vi "Main.vi"(8 "error in (no error)":errorcluster) -> ()   [LabVIEW 2017, in "EventModule.lvlib"]
uses:
  EventModule.lvlib
  <userlib>/NIST/ModuleAdminLib/ModuleAdmin/ModuleAdmin.lvclass
  C:/Program Files (x86)/National Instruments/LabVIEW 2017/user.lib/NIST/ModuleAdminLib/ModuleAdminBase/ModuleAdminBase.lvclass
  PublicAPI/Arguments/Requests/clStopArgument.ctl
  EventPlugins/EventPluginBaseClass/EventPluginBaseClass.lvclass
  C:/Program Files (x86)/National Instruments/LabVIEW 2017/user.lib/NIST/BaseClasses/BasePlugin_class/BasePlugin.lvclass
  <userlib>/NIST/ModuleAdminLib/ModuleAdmin/ModuleAdmin.lvclass/ModuleAdmin.ctl
  <userlib>/NIST/BaseClasses/BasePlugin_class/BasePlugin.lvclass/BasePlugin.ctl
  EventPlugins/EventPluginBaseClass/TypeDefs/clEvtConfig.ctl
  PublicAPI/Arguments/Requests/dblTimeArray.ctl
  PublicAPI/Arguments/Requests/dblEvtParams.ctl
  EventPlugins/EventPluginBaseClass/EventPluginBaseClass.lvclass/EventPluginBaseClass.ctl
  <vilib>/Utility/error.llb/DialogType.ctl
  <userlib>/NIST/ModuleAdminLib/ModuleAdmin/Accessors/Read ShowPanel_.vi
  <userlib>/NIST/ModuleAdminLib/ModuleAdmin/Accessors/Write ShowPanel_.vi
  <userlib>/NIST/BaseClasses/BasePlugin_class/Accessors/Write PluginIniFilePath.vi
  <userlib>/NIST/BaseClasses/BasePlugin_class/Accessors/Read PluginIniFilePath.vi
  EventPlugins/EventPluginBaseClass/Accessors/Write BusNumber.vi
  EventPlugins/EventPluginBaseClass/Accessors/Read BusNumber.vi
  <userlib>/NIST/ModuleAdminLib/ModuleAdmin/Accessors/Read CloneRegRef.vi
  <vilib>/Utility/error.llb/Error Cluster From Error Code.vi
  EventPlugins/EventPluginBaseClass/Accessors/Write EvtConfig.vi
  EventPlugins/EventPluginBaseClass/Accessors/Read EvtConfig.vi
  <vilib>/Analysis/1siggen.llb/Ramp Pattern by Delta.vi
  EventPlugins/EventPluginBaseClass/Accessors/Read TimeArray.vi
  EventPlugins/EventPluginBaseClass/Accessors/Read EvtParams.vi
  <vilib>/ErrorRing/Error Ring.xnode
  <userlib>/NIST/ModuleAdminLib/CloneRegistration/CloneRegistration.lvclass
  <userlib>/NIST/ModuleAdminLib/ModuleAdmin.lvlib
  <userlib>/NIST/BaseClasses/Object_class/BaseObject.lvclass
  <vilib>/Analysis/NI_AALBase.lvlib
panel:
  out "error out":errorcluster
  in  "ModuleAdmin":refnum<class "ModuleAdmin.lvclass">
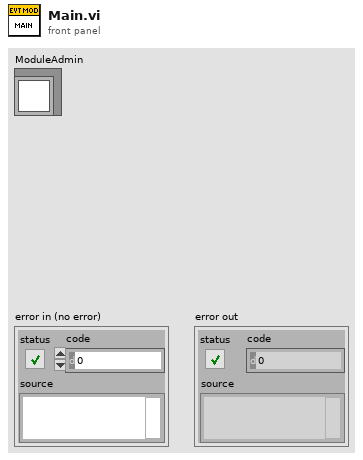
[diagram p1: front panel]
types:
  T1 = typedef "EventModule.lvlib/clRequestEvents.ctl" = cluster{"StopRequest":refnum<user-event>, "LoadPluginRequest":refnum<user-event>, "WriteEvtConfig":refnum<user-event>, "ReadEvtConfig":refnum<user-event>, "WriteTimeArray":refnum<user-event>, "ReadTimeArray":refnum<user-event>, "WriteEvtParams":refnum<user-event>, "ReadEvtParams":refnum<user-event>, "GetEvtReportArray":refnum<user-event>, "ReadPathToPlugin":refnum<user-event>, "GetEvtSignal":refnum<user-event>, "WriteBusNumber":refnum<user-event>, "ReadBusNumber":refnum<user-event>, "ShowPanel":refnum<user-event>}
  T2 = typedef "EventModule.lvlib/clBroadcastEvents.ctl" = cluster{"DidInit":refnum<user-event>, "StatusUpdate":refnum<user-event>, "ErrorReport":refnum<user-event>, "DidStop":refnum<user-event>, "ReadEvtConfig":refnum<user-event>, "ReadTimeArray":refnum<user-event>, "ReadEvtParams":refnum<user-event>, "GetEvtReportArray":refnum<user-event>, "ReadPathToPlugin":refnum<user-event>, "GetEvtSignal":refnum<user-event>, "ReadBusNumber":refnum<user-event>}
  T3 = typedef "EventModule.lvlib/clStopArgument.ctl" = cluster{"Exit via Stop Module Req?":bool, "Wait for Module to stop?":bool, "ModuleAdmin":refnum<class "ModuleAdmin.lvclass">}
  T4 = enum32{"Invalid", "Standard", "Closed", "Hidden", "Minimized", "Maximized"}
  T5 = typedef "EventPlugins.lvlib/EventPluginBaseClass.lvclass/clEvtConfig.ctl" = cluster{"T0(UTC)":dbl, "F0":dbl, "Fs":i32, "FSamp":u32, "bPosSeq":bool}
  T6 = typedef "EventModule.lvlib/dblTimeArray.ctl" = dbl[]
  T7 = typedef "EventModule.lvlib/dblEvtParams.ctl" = dbl[][]
  T8 = typedef "EventPlugins.lvlib/EventPluginBaseClass.lvclass/clEvtReportArray.ctl" = T9[]
  T9 = typedef "EventPlugins.lvlib/EventPluginBaseClass.lvclass/clEvtReport.ctl" = cluster{"Timestamp":dbl, "Synx":cdb[], "Freq":dbl, "ROCOF":dbl, "ID":i16}
  T10 = typedef "EventPlugins.lvlib/EventPluginBaseClass.lvclass/dblEvtSignalArray.ctl" = dbl[][]
  T11 = typedef "DialogType.ctl" = u16
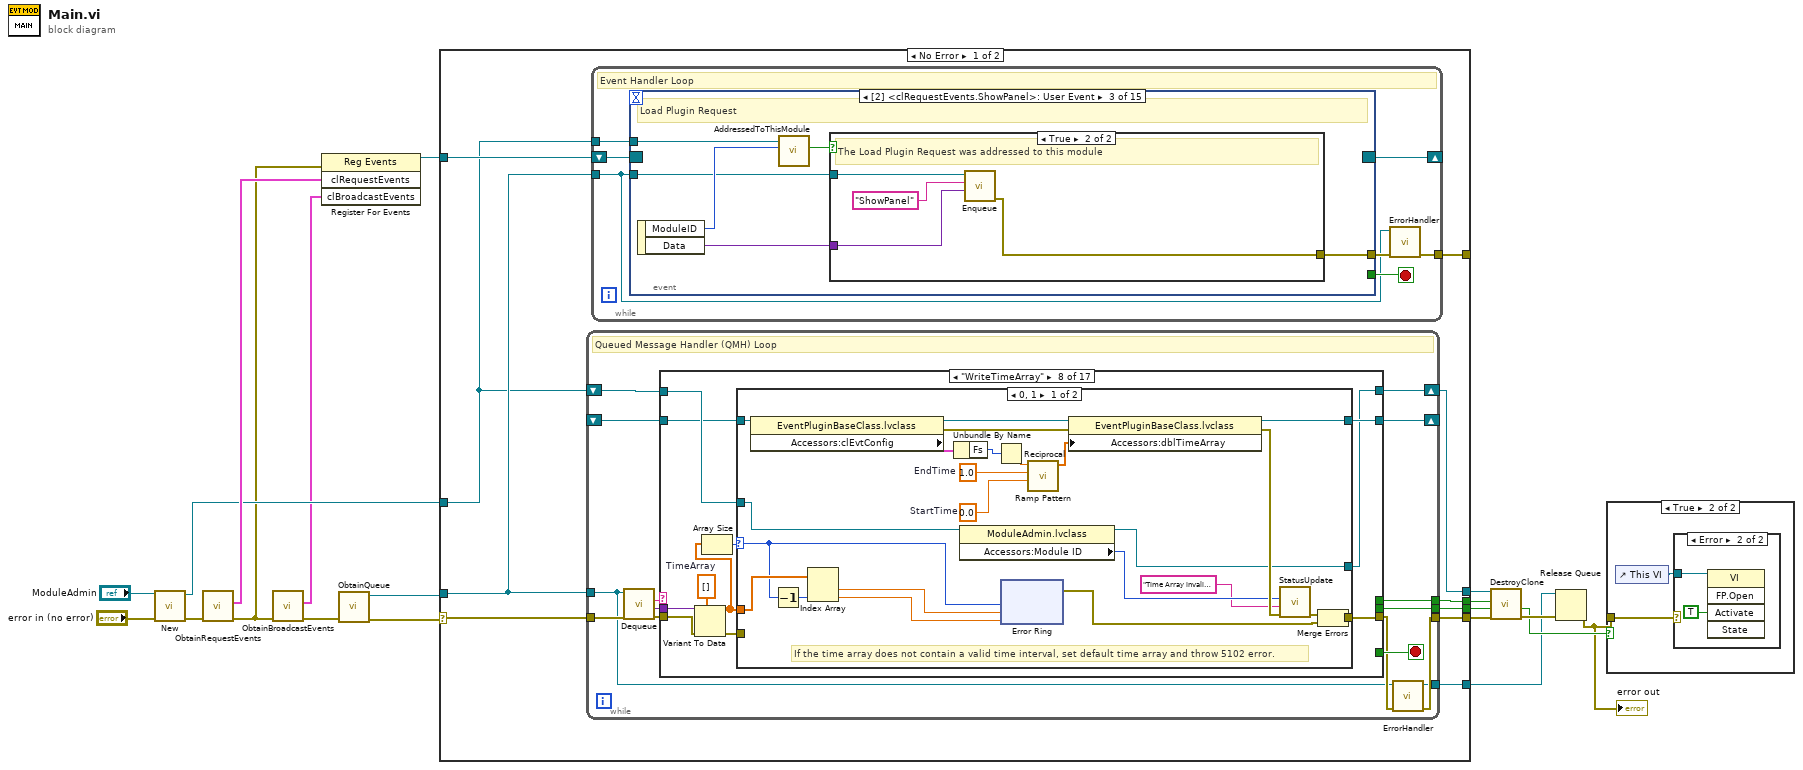
[diagram p0: block diagram]
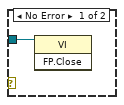
[diagram p3: hidden frame]
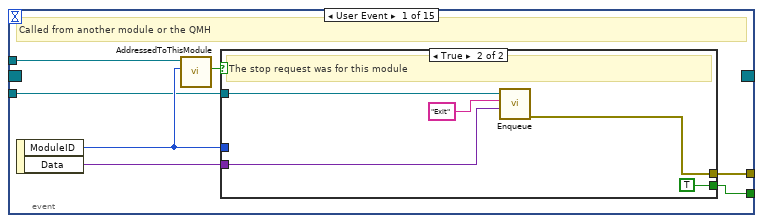
[diagram p4: hidden frame]
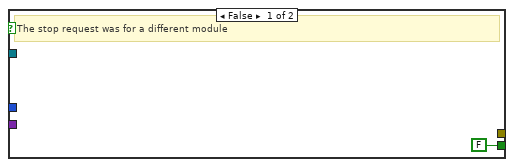
[diagram p5: hidden frame]
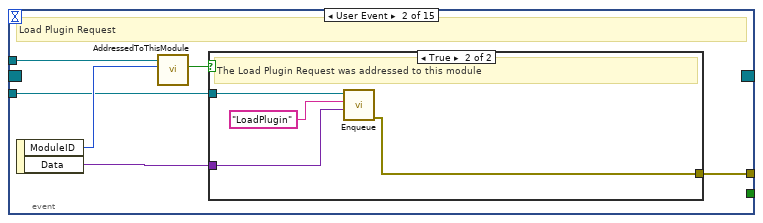
[diagram p6: hidden frame]
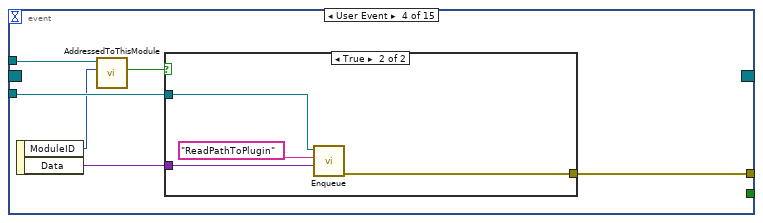
[diagram p9: hidden frame]
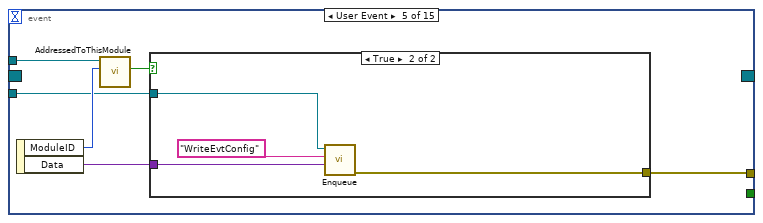
[diagram p11: hidden frame]
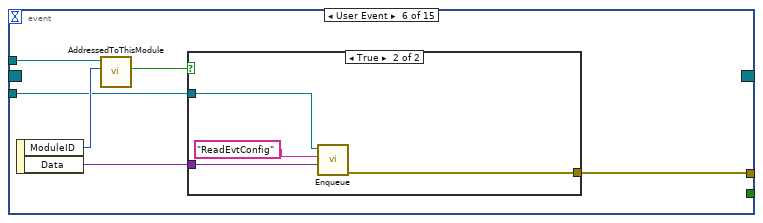
[diagram p13: hidden frame]
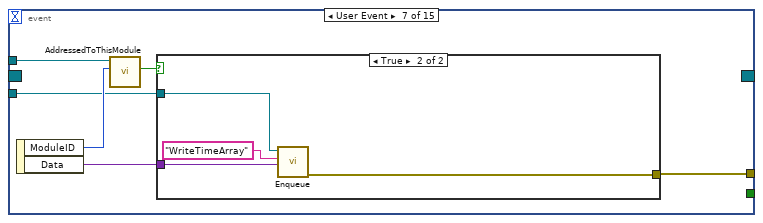
[diagram p15: hidden frame]
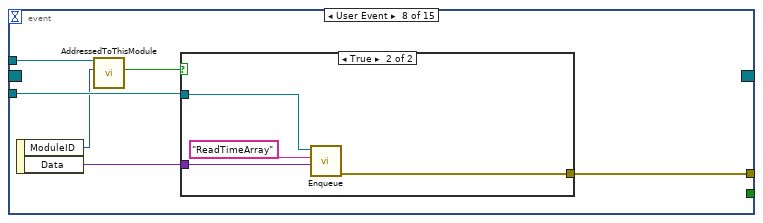
[diagram p17: hidden frame]
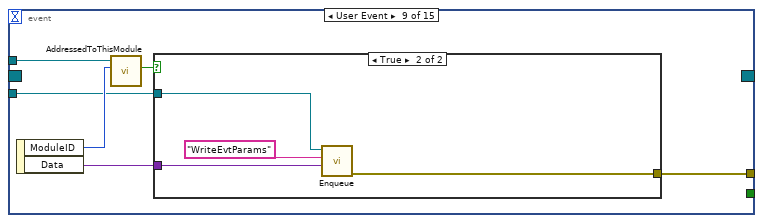
[diagram p19: hidden frame]
diagram:
  n1 = call <userlib>:"New.vi"("error in (no error)"="error in (no error)", "ModuleAdmin"="ModuleAdmin") -> ("error out"=w17:errorcluster, "ModuleAdmin"=w13:refnum<class "ModuleAdmin.lvclass">)  [unwired: 7 in, 1 out]
  n2 = call "ObtainRequestEvents.vi"("error in (no error)"=w17) -> ("error out"=w11:errorcluster, "clRequestEvents"=w16:T1)  [unwired: 9 in]
  n3 = call "ObtainBroadcastEvents.vi"("error in (no error)"=w11) -> ("error out"=w12:errorcluster, "clBroadcastEvents"=w10:T2)  [unwired: 9 in]
  n4 = register-events(error in=w11, w16, w10) -> (reference out=w9:refnum<event-registration>)  [unwired: 1 in, 1 out]
  n5 = call "ObtainQueue.vi"("error in (no error)"=w12) -> ("error out"=w15:errorcluster, "MessageQueue"=w14:refnum<queue>)  [unwired: 9 in]
  n6 = case shown="No Error" w15 {
    selector: w15 -> [w29 w509]
    tunnel: w14 -> [w27 w504]
    tunnel: w13 -> [w25 w506]
    tunnel: [w28 w507] -> w8
    tunnel: w9 -> [w26 _]
    tunnel: [w20 w505] -> w6
    tunnel: [w24 _] -> w5
    tunnel: [w23 _] -> w4
    tunnel: [w22 _] -> _
    tunnel: [w21 w504] -> w1
    frame No Error {
      n7 = while {
        tunnel: w27 -> [w197]
        tunnel: w29 -> [w206]
        tunnel: [w199] -> w28
        tunnel: [w201] -> w24
        tunnel: [w200] -> w23
        tunnel: [w196] -> w21
        shift-right: [w195] -> _
        shift-left: _ -> [w194]
        shift-right: [w193] -> w20
        shift-left: w25 -> [w202]
        stop <- w207 stop-if-true
        # "Queued Message Handler (QMH) Loop"
        n8 = call "Dequeue.vi"("error in (no error)"=w206, "MessageQueue"=w197) -> ("error out"=w205:errorcluster, "Message Data"=w203:variant, "Message"=w204:string)  [unwired: 6 in, 1 out]
        n9 = case shown="\"WriteTimeArray\"" w204 {
          selector: w204 -> [w212 _ _ _ _ _ _ _ _ _ _ _ _ _ _ _ _]
          tunnel: [_ _ _ _ _ _ _ _ _ _ _ _ _ _ _ TRUE _] -> w207
          tunnel: w202 -> [w215 w244 w263 w267 w317 w327 w342 w352 w400 w410 w424 w435 w444 w462 w475 w476 w496]
          tunnel: [w211 w233 w254 w268 w312 w329 w336 w351 w399 w409 w423 w434 w443 w452 w465 w483 w487] -> w198
          tunnel: w205 -> [_ _ w260 w279 w316 w331 w339 w353 w401 w411 w425 w436 w445 w461 w474 w482 w495]
          tunnel: w203 -> [_ _ w259 w282 _ w332 _ w354 _ w412 w426 _ _ _ _ w481 w494]
          tunnel: [_ _ _ _ _ _ _ _ _ _ _ _ _ _ _ w479 _] -> w201
          tunnel: [_ _ _ _ _ _ _ _ _ _ _ _ _ _ _ w478 _] -> w200
          tunnel: [w209 refnum<class "EventPluginBaseClass.lvclass"> refnum ("EventPlugins.lvlib:EventPluginBaseClass.lvclass") w264 w273 w315 w328 w341 w349 w402 w407 w421 w433 w442 w458 w471 w477 w486] -> w195
          tunnel: w194 -> [w209 _ w264 w274 w318 w322 w343 w348 w403 w408 w422 w437 w446 w460 w473 w477 w486]
          tunnel: [w208 w224 w262 w265 w309 w320 w333 w344 w397 w406 w419 w432 w441 w450 w463 w476 w485] -> w193
          frame Default {
            n10 = property class="ModuleAdmin.lvclass"(reference=w215) -> (reference out=w208:refnum<class "ModuleAdmin.lvclass">, "Accessors:Module ID"=w214:i32, "Accessors:ModuleName"=w210:string)  [unwired: 1 in, 1 out]
            n11 = call <userlib>:"ModuleName.vi"("Name"=w210, "ModuleID"=w214) -> ("ModuleName"=w213:string)  [unwired: 9 in]
            n12 = xnode "Error Ring"("parameter 0"=w212, "parameter 1"=w213) -> ("error out"=w211:errorcluster)
          }
          frame "Initialize" {
            n13 = property class="ModuleAdmin.lvclass"(reference=w244) -> (reference out=w229:refnum<class "ModuleAdmin.lvclass">, error out=w241:errorcluster, "Accessors:Module ID"=w232:i32, "Accessors:ShowPanel_"=w227:bool, "Accessors:External Launch"=w226:bool, "Accessors:ModuleName"=w228:string)  [unwired: 1 in]
            n14 = Compound Arithmetic op=OR(w227, invert w226) -> (w225:bool)
            n15 = Select(t=T4."Standard" ("Front Panel Window:State"), s=w225, f=T4."Hidden" ("Front Panel Window:State")) -> (s? t:f=w237:T4)
            n16 = invoke class="VI" method="FP.Open"(error in=w241, "State"=w237) -> (error out=w240:errorcluster)  [unwired: 3 in, 4 out]
            n17 = call <userlib>:"ModuleName.vi"("Name"=w228, "ModuleID"=w232) -> ("ModuleName"=w236:string)  [unwired: 9 in]
            n18 = property class="VI"(error in=w240, "Front Panel.Title"=w236) -> (reference out=w243:refnum<vi>, error out=w242:errorcluster)  [unwired: 1 in]
            n19 = invoke class="VI" method="FP.Center"(reference=w243, error in=w242) -> (error out=w231:errorcluster)  [unwired: 1 in, 2 out]
            n20 = case shown="True" w226 {
              tunnel: [w245 w251] -> w234
              tunnel: [w246 w248] -> w224
              tunnel: w231 -> [w245 w250]
              tunnel: w229 -> [w246 w247]
              frame False {
              }
              frame True {
                n21 = call <userlib>:"WaitOnModuleSync.vi"("error in (no error)"=w250, "ModuleAdmin"=w247) -> ("error out"=w252:errorcluster, "ModuleAdmin"=w249:refnum<class "ModuleAdmin.lvclass">)  [unwired: 8 in]
                n22 = call <userlib>:"WaitOnEventSync.vi"("error in (no error)"=w252, "ModuleAdmin"=w249) -> ("error out"=w251:errorcluster, "ModuleAdmin"=w248:refnum<class "ModuleAdmin.lvclass">)  [unwired: 8 in]
              }
            }
            n23 = call "DidInit.vi"("Init?"=TRUE, "error in (no error)"=w234, "ModuleAdmin"=w224) -> ("error out"=w233:errorcluster)  [unwired: 8 in]
          }
          frame "ShowPanel" {
            n24 = Variant To Data(error in=w260, type=FALSE, Variant=w259) -> (data=w253:bool, error out=w258:errorcluster)
            n25 = Select(t=T4."Standard" ("Front Panel Window:State"), s=w253, f=T4."Hidden" ("Front Panel Window:State")) -> (s? t:f=w255:T4)
            n26 = property class="VI"(error in=w258, "FP.State"=w255) -> (error out=w254:errorcluster)  [unwired: 1 in, 1 out]
            n27 = property class="ModuleAdmin.lvclass"(reference=w263, "Accessors:ShowPanel_"=w253) -> (reference out=w262:refnum<class "ModuleAdmin.lvclass">)  [unwired: 1 in, 1 out]
          }
          frame "LoadPlugin" {
            n28 = Variant To Data(error in=w279, type=path "", Variant=w282) -> (data=w266:path, error out=w280:errorcluster)
            n29 = call <userlib>:"GetPathToClass.vi"("error in (no error)"=w280, "configuration file path"=w266) -> ("error IO"=w278:errorcluster, "PathToClass"=w269:path)  [unwired: 8 in]
            n30 = Current VI's Path() -> (path=w270:path)
            n31 = Build Path(base path=w270, name or relative path=w269) -> (appended path=w271:path)
            n32 = call <vilib>:"Check if File or Folder Exists.vi"("error in (no error)"=w278, "path"=w271) -> ("error out"=w276:errorcluster, "file or folder exists?"=w277:bool, "dup path"=w275:path)  [unwired: 7 in]
            n33 = case shown="True" w277 {
              tunnel: w275 -> [w290 w296]
              tunnel: w276 -> [w294 w299]
              tunnel: [w288 w300] -> w268
              tunnel: w274 -> [_ w301]
              tunnel: [w289 w301] -> w272
              tunnel: w267 -> [w284 w295]
              tunnel: [w283 w295] -> w265
              frame True {
                n34 = call-dynamic "LoadClassFromFile.vi"("error in (no error)"=w294, "class path"=w290, "reference in"=refnum<class "EventPluginBaseClass.lvclass"> refnum ("EventPlugins.lvlib:EventPluginBaseClass.lvclass")) -> ("error out"=w287:errorcluster, "reference out"=w289:refnum<class "EventPluginBaseClass.lvclass">)  [unwired: 7 in]
                n35 = property class="ModuleAdmin.lvclass"(reference=w284) -> (reference out=w283:refnum<class "ModuleAdmin.lvclass">, "Accessors:Module ID"=w285:i32)  [unwired: 1 in, 1 out]
                n36 = Path To String(path=w290) -> (string=w292:string)
                n37 = Format Into String(format string="Plugin %s loaded", w292) -> (resulting string=w286:string)  [unwired: 2 in, 1 out]
                n38 = call "StatusUpdate.vi"("error in (no error)"=w287, "Status"=w286, "ModuleID"=w285) -> ("error out"=w288:errorcluster)  [unwired: 8 in]
              }
              frame False {
                n39 = Path To String(path=w296) -> (string=w297:string)
                n40 = xnode "Error Ring"("parameter 0"=w297) -> ("error out"=w298:errorcluster)
                n41 = Merge Errors(w298, w299) -> (w300:errorcluster)
              }
            }
            n42 = property class="EventPluginBaseClass.lvclass"(reference=w272, "Accessors:PluginIniFilePath"=w266) -> (reference out=w273:refnum<class "EventPluginBaseClass.lvclass">)  [unwired: 1 in, 1 out]
          }
          frame "ReadPathToPlugin" {
            n43 = property class="EventPluginBaseClass.lvclass"(reference=w318, error in=w316) -> (reference out=w315:refnum<class "EventPluginBaseClass.lvclass">, error out=w319:errorcluster, "Accessors:PluginIniFilePath"=w314:path)
            n44 = property class="ModuleAdmin.lvclass"(reference=w317) -> (reference out=w309:refnum<class "ModuleAdmin.lvclass">, "Accessors:Module ID"=w311:i32)  [unwired: 1 in, 1 out]
            n45 = call "ReadPathToPlugin.vi"("error in (no error)"=w319, "EvtPluginINIFilePath"=w314, "ModuleID"=w311) -> ("error out"=w313:errorcluster)  [unwired: 8 in]
            n46 = call "StatusUpdate.vi"("error in (no error)"=w313, "Status"="PathToPlugin Transmitted", "ModuleID"=w311) -> ("error out"=w312:errorcluster)  [unwired: 8 in]
          }
          frame "WriteEvtConfig" {
            n47 = Variant To Data(error in=w331, type=T5 {"T0(UTC)"=0.0, "F0"=0.0, "Fs"=0, "FSamp"=0, "bPosSeq"=FALSE} ("clEvtConfig"), Variant=w332) -> (data=w323:T5, error out=w321:errorcluster)
            n48 = property class="EventPluginBaseClass.lvclass"(reference=w322, error in=w321, "Accessors:clEvtConfig"=w323) -> (reference out=w328:refnum<class "EventPluginBaseClass.lvclass">, error out=w324:errorcluster)
            n49 = property class="ModuleAdmin.lvclass"(reference=w327) -> (reference out=w320:refnum<class "ModuleAdmin.lvclass">, "Accessors:Module ID"=w326:i32)  [unwired: 1 in, 1 out]
            n50 = call "StatusUpdate.vi"("error in (no error)"=w324, "Status"="Event Configuration Received", "ModuleID"=w326) -> ("error out"=w329:errorcluster)  [unwired: 8 in]
          }
          frame "ReadEvtConfig" {
            n51 = property class="EventPluginBaseClass.lvclass"(reference=w343, error in=w339) -> (reference out=w341:refnum<class "EventPluginBaseClass.lvclass">, error out=w340:errorcluster, "Accessors:clEvtConfig"=w338:T5)
            n52 = property class="ModuleAdmin.lvclass"(reference=w342) -> (reference out=w333:refnum<class "ModuleAdmin.lvclass">, "Accessors:Module ID"=w335:i32)  [unwired: 1 in, 1 out]
            n53 = call "ReadEvtConfig.vi"("error in (no error)"=w340, "clEvtConfigReport"=w338, "ModuleID"=w335) -> ("error out"=w337:errorcluster)  [unwired: 8 in]
            n54 = call "StatusUpdate.vi"("error in (no error)"=w337, "Status"="Evt Config Transmitted", "ModuleID"=w335) -> ("error out"=w336:errorcluster)  [unwired: 8 in]
          }
          frame "WriteTimeArray" {
            w350 = T6 []  # TimeArray
            n55 = Variant To Data(error in=w353, type=w350, Variant=w354) -> (data=w345:T6, error out=w347:errorcluster)
            n56 = Array Size(array=w345) -> (size(s)=w346:i32)
            n57 = case shown="0, 1" w346 {
              selector: w346 -> [w357 _]
              tunnel: w352 -> [w367 w395]
              tunnel: [w370 w394] -> w351
              tunnel: [w377 w393] -> w349
              tunnel: w348 -> [w376 w390]
              tunnel: w347 -> [_ w389]
              tunnel: w345 -> [w359 w388]
              tunnel: [w360 w387] -> w344
              frame 0, 1 {
                w373 = 0.0  # StartTime
                w374 = 1.0  # EndTime
                # "If the time array does not contain a valid time interval, set default time array and throw 5102 error."
                n58 = property class="EventPluginBaseClass.lvclass"(reference=w376) -> (reference out=w375:refnum<class "EventPluginBaseClass.lvclass">, error out=w372:errorcluster, "Accessors:clEvtConfig"=w363:T5)  [unwired: 1 in]
                n59 = Decrement(x=w357) -> (x-1=w358:i32)
                n60 = Index Array(array=w359, index #2=w358) -> (element #1=w356:dbl, element #2=w355:dbl)  [unwired: 1 in]
                n61 = Unbundle By Name(w363) -> ("Fs"=w362:i32)
                n62 = property class="ModuleAdmin.lvclass"(reference=w367) -> (reference out=w360:refnum<class "ModuleAdmin.lvclass">, "Accessors:Module ID"=w366:i32)  [unwired: 1 in, 1 out]
                n63 = Reciprocal(x=w362) -> (1/x=w364:dbl)
                n64 = xnode "Error Ring"("parameter 0"=w357, "parameter 1"=w356, "parameter 2"=w355) -> ("error out"=w369:errorcluster)
                n65 = call-poly <vilib>:"Ramp Pattern.vi"("start"=w373, "end"=w374, "delta"=w364) -> ("Ramp Pattern"=w361:dbl[])  [unwired: 6 in, 2 out]
                n66 = property class="EventPluginBaseClass.lvclass"(reference=w375, error in=w372, "Accessors:dblTimeArray"=w361) -> (reference out=w377:refnum<class "EventPluginBaseClass.lvclass">, error out=w368:errorcluster)
                n67 = call "StatusUpdate.vi"("error in (no error)"=w368, "Status"="Time Array invalid, setting 0 to 1 sec interval", "ModuleID"=w366) -> ("error out"=w371:errorcluster)  [unwired: 8 in]
                n68 = Merge Errors(w371, w369) -> (w370:errorcluster)
              }
              frame Default {
                n69 = property class="ModuleAdmin.lvclass"(reference=w395) -> (reference out=w387:refnum<class "ModuleAdmin.lvclass">, "Accessors:Module ID"=w391:i32)  [unwired: 1 in, 1 out]
                n70 = property class="EventPluginBaseClass.lvclass"(reference=w390, error in=w389, "Accessors:dblTimeArray"=w388) -> (reference out=w393:refnum<class "EventPluginBaseClass.lvclass">, error out=w392:errorcluster)
                n71 = call "StatusUpdate.vi"("error in (no error)"=w392, "Status"="Time Array Received", "ModuleID"=w391) -> ("error out"=w394:errorcluster)  [unwired: 8 in]
              }
            }
          }
          frame "ReadTimeArray" {
            n72 = property class="EventPluginBaseClass.lvclass"(reference=w403, error in=w401) -> (reference out=w402:refnum<class "EventPluginBaseClass.lvclass">, error out=w404:errorcluster, "Accessors:dblTimeArray"=w398:dbl[])
            n73 = property class="ModuleAdmin.lvclass"(reference=w400) -> (reference out=w397:refnum<class "ModuleAdmin.lvclass">, "Accessors:Module ID"=w405:i32)  [unwired: 1 in, 1 out]
            n74 = call "ReadTimeArray.vi"("error in (no error)"=w404, "dblTime Array"=w398, "ModuleID"=w405) -> ("error out"=w399:errorcluster)  [unwired: 8 in]
          }
          frame "WriteEvtParams" {
            w413 = T7 []  # SignalParams
            # "Can't change \"SignalParams\" to icon."
            n75 = Variant To Data(error in=w411, type=w413, Variant=w412) -> (data=w414:T7, error out=w418:errorcluster)
            n76 = property class="EventPluginBaseClass.lvclass"(reference=w408, error in=w418, "Accessors:dblEvtParams"=w414) -> (reference out=w407:refnum<class "EventPluginBaseClass.lvclass">, error out=w415:errorcluster)
            n77 = property class="ModuleAdmin.lvclass"(reference=w410) -> (reference out=w406:refnum<class "ModuleAdmin.lvclass">, "Accessors:Module ID"=w417:i32)  [unwired: 1 in, 1 out]
            n78 = call "StatusUpdate.vi"("error in (no error)"=w415, "Status"="Event Parameters Received", "ModuleID"=w417) -> ("error out"=w409:errorcluster)  [unwired: 8 in]
          }
          frame "WriteBusNumber" {
            n79 = Variant To Data(error in=w425, type=u8 0, Variant=w426) -> (data=w427:u8, error out=w431:errorcluster)
            n80 = property class="EventPluginBaseClass.lvclass"(reference=w422, error in=w431, "Accessors:BusNumber"=w427) -> (reference out=w421:refnum<class "EventPluginBaseClass.lvclass">, error out=w428:errorcluster)
            n81 = property class="ModuleAdmin.lvclass"(reference=w424) -> (reference out=w419:refnum<class "ModuleAdmin.lvclass">, "Accessors:Module ID"=w430:i32)  [unwired: 1 in, 1 out]
            n82 = call "StatusUpdate.vi"("error in (no error)"=w428, "Status"="Bus Number Received", "ModuleID"=w430) -> ("error out"=w423:errorcluster)  [unwired: 8 in]
          }
          frame "ReadEvtParams" {
            n83 = property class="EventPluginBaseClass.lvclass"(reference=w437, error in=w436) -> (reference out=w433:refnum<class "EventPluginBaseClass.lvclass">, error out=w439:errorcluster, "Accessors:dblEvtParams"=w438:dbl[][])
            n84 = property class="ModuleAdmin.lvclass"(reference=w435) -> (reference out=w432:refnum<class "ModuleAdmin.lvclass">, "Accessors:Module ID"=w440:i32)  [unwired: 1 in, 1 out]
            n85 = call "ReadEvtParams.vi"("error in (no error)"=w439, "SignalParams"=w438, "ModuleID"=w440) -> ("error out"=w434:errorcluster)  [unwired: 8 in]
          }
          frame "ReadBusNumber" {
            n86 = property class="EventPluginBaseClass.lvclass"(reference=w446, error in=w445) -> (reference out=w442:refnum<class "EventPluginBaseClass.lvclass">, error out=w448:errorcluster, "Accessors:BusNumber"=w447:u8)
            n87 = property class="ModuleAdmin.lvclass"(reference=w444) -> (reference out=w441:refnum<class "ModuleAdmin.lvclass">, "Accessors:Module ID"=w449:i32)  [unwired: 1 in, 1 out]
            n88 = call "ReadBusNumber.vi"("error in (no error)"=w448, "BusNumber"=w447, "ModuleID"=w449) -> ("error out"=w443:errorcluster)  [unwired: 8 in]
          }
          frame "GetReportArray" {
            n89 = call-dynamic "GetEvtReports.vi"("error in (no error)"=w461, "EventPluginBaseClass in"=w460) -> ("error out"=w457:errorcluster, "EventPluginBaseClass out"=w459:refnum<class "EventPluginBaseClass.lvclass">)  [unwired: 8 in]
            n90 = property class="EventPluginBaseClass.lvclass"(reference=w459, error in=w457) -> (reference out=w458:refnum<class "EventPluginBaseClass.lvclass">, error out=w456:errorcluster, "Accessors:clEvtReportArray"=w455:T8)
            n91 = property class="ModuleAdmin.lvclass"(reference=w462) -> (reference out=w450:refnum<class "ModuleAdmin.lvclass">, "Accessors:Module ID"=w451:i32)  [unwired: 1 in, 1 out]
            n92 = call "GetEvtReports.vi"("error in (no error)"=w456, "clReportArray"=w455, "ModuleID"=w451) -> ("error out"=w453:errorcluster)  [unwired: 8 in]
            n93 = call "StatusUpdate.vi"("error in (no error)"=w453, "Status"="Event Reports Transmitted", "ModuleID"=w451) -> ("error out"=w452:errorcluster)  [unwired: 8 in]
          }
          frame "GetEvtSignal" {
            n94 = call-dynamic "GetEvtSignal.vi"("error in (no error)"=w474, "EventPluginBaseClass in"=w473) -> ("error out"=w470:errorcluster, "EventPluginBaseClass out"=w472:refnum<class "EventPluginBaseClass.lvclass">)  [unwired: 8 in]
            n95 = property class="EventPluginBaseClass.lvclass"(reference=w472, error in=w470) -> (reference out=w471:refnum<class "EventPluginBaseClass.lvclass">, error out=w469:errorcluster, "Accessors:dblEventSignalArray"=w468:T10)
            n96 = property class="ModuleAdmin.lvclass"(reference=w475) -> (reference out=w463:refnum<class "ModuleAdmin.lvclass">, "Accessors:Module ID"=w464:i32)  [unwired: 1 in, 1 out]
            n97 = call "GetEvtSignal.vi"("error in (no error)"=w469, "clReportArray"=w468, "ModuleID"=w464) -> ("error out"=w466:errorcluster)  [unwired: 8 in]
            n98 = call "StatusUpdate.vi"("error in (no error)"=w466, "Status"="Event Signal Transmitted", "ModuleID"=w464) -> ("error out"=w465:errorcluster)  [unwired: 8 in]
          }
          frame "Exit" {
            n99 = control-ref of="This VI"() -> (w480:refnum<vi>)
            n100 = call "HandleExit.vi"("error in (no error)"=w482, "VI Refnum"=w480, "StopArgument"=w481, "ModuleAdmin"=w476) -> ("error out"=w483:errorcluster, "Exit via Stop Module Req?"=w478:bool, "WaitForStop?"=w479:bool)  [unwired: 5 in]
          }
          frame "Error" {
            n101 = property class="ModuleAdmin.lvclass"(reference=w496) -> (reference out=w485:refnum<class "ModuleAdmin.lvclass">, "Accessors:External Launch"=w490:bool, "Accessors:Module ID"=w488:i32)  [unwired: 1 in, 1 out]
            n102 = Variant To Data(error in=w495, type=errorcluster {"status"=FALSE, "code"=0, "source"=""} ("error constant"), Variant=w494) -> (data=w489:errorcluster, error out=w492:errorcluster)
            n103 = call "ReportError.vi"("error in (no error)"=w492, "ErrorReported"=w489, "ModuleID"=w488) -> ("error out"=w491:errorcluster)  [unwired: 8 in]
            n104 = case shown="True" w490 {
              tunnel: w491 -> [w500 w501]
              tunnel: w489 -> [w499 _]
              tunnel: [w498 w501] -> w487
              tunnel: w485 -> [w497 _]
              frame False {
                # "Todo:  Add an event to ask the user\nIf the module should stop or continue"
                # "Stand alone: now, force an exit"
                n105 = call <vilib>:"Simple Error Handler.vi"("error in (no error)"=w499) -> ()  [unwired: 4 in, 5 out]
                n106 = call "StopRequest.vi"("error in (no error)"=w500, "ModuleAdmin"=w497) -> ("error out"=w498:errorcluster)  [unwired: 8 in, 1 out]
              }
              frame True {
                # "Externally launched modules only broadcast the error msg"
              }
            }
          }
        }
        n107 = call "ErrorHandler.vi"("error in (no error)"=w198, "MessageQueue"=w197) -> ("error out"=w199:errorcluster, "MessageQueue"=w196:refnum<queue>)  [unwired: 8 in]
      }
      n108 = while {
        tunnel: w27 -> [w30]
        shift-right: [w34] -> _
        shift-left: w26 -> [w35]
        tunnel: w25 -> [w33]
        tunnel: [w31] -> w22
        stop <- w36 stop-if-true
        # "Event Handler Loop"
        n109 = event shown="[2] <clRequestEvents.ShowPanel>: User Event" {
          selector: w35 -> [_ _ _ _ _ _ _ _ _ _ _ _ _ _ _]
          dyn-events: [_ _ _ _ _ _ _ _ _ _ _ _ _ _ _] -> w34
          timeout: _ -> [_ _ _ _ _ _ _ _ _ _ _ _ _ _ _]
          tunnel: w30 -> [w40 w53 w63 w73 w81 w91 w100 w113 w121 w131 w141 w151 w162 w172 w192]
          tunnel: [w39 _ _ _ _ _ _ _ _ _ _ _ _ _ TRUE] -> w36
          tunnel: w33 -> [w43 w51 w61 w74 w84 w95 w103 w114 w122 w133 w142 w152 w164 w174 w186]
          tunnel: [w38 w52 w62 w70 w80 w90 w104 w110 w120 w130 w140 w150 w160 w170 w190] -> w32
          event User Event {
            # "Called from another module or the QMH"
            n110 = event-data() -> ("ModuleID"=w41:i32, "Data"=w37:variant)  [unwired: 1 in]
            n111 = call <userlib>:"AddressedToThisModule.vi"("ModuleID"=w41, "ModuleAdmin"=w43) -> ("AddressedToThisInstance?"=w42:bool)  [unwired: 8 in, 1 out]
            n112 = case shown="True" w42 {
              tunnel: w41 -> [_ _]
              tunnel: w40 -> [_ w49]
              tunnel: [FALSE TRUE] -> w39
              tunnel: [_ w47] -> w38
              tunnel: w37 -> [_ w45]
              frame False {
                # "The stop request was for a different module"
              }
              frame True {
                # "The stop request was for this module"
                n113 = call "Enqueue.vi"("Message Data"=w45, "Message"="Exit", "MessageQueue"=w49) -> ("error out"=w47:errorcluster)  [unwired: 7 in, 1 out]
              }
            }
          }
          event User Event {
            # "Load Plugin Request"
            n114 = event-data() -> ("ModuleID"=w54:i32, "Data"=w50:variant)  [unwired: 1 in]
            n115 = call <userlib>:"AddressedToThisModule.vi"("ModuleID"=w54, "ModuleAdmin"=w51) -> ("AddressedToThisInstance?"=w55:bool)  [unwired: 8 in, 1 out]
            n116 = case shown="True" w55 {
              tunnel: w50 -> [_ w59]
              tunnel: w53 -> [_ w58]
              tunnel: [_ w56] -> w52
              frame False {
                # "Not addressed to this module"
              }
              frame True {
                # "The Load Plugin Request was addressed to this module"
                n117 = call "Enqueue.vi"("Message Data"=w59, "Message"="LoadPlugin", "MessageQueue"=w58) -> ("error out"=w56:errorcluster)  [unwired: 7 in, 1 out]
              }
            }
          }
          event User Event {
            # "Load Plugin Request"
            n118 = event-data() -> ("ModuleID"=w64:i32, "Data"=w60:variant)  [unwired: 1 in]
            n119 = call <userlib>:"AddressedToThisModule.vi"("ModuleID"=w64, "ModuleAdmin"=w61) -> ("AddressedToThisInstance?"=w65:bool)  [unwired: 8 in, 1 out]
            n120 = case shown="True" w65 {
              tunnel: w60 -> [_ w69]
              tunnel: w63 -> [_ w68]
              tunnel: [_ w66] -> w62
              frame False {
                # "Not addressed to this module"
              }
              frame True {
                # "The Load Plugin Request was addressed to this module"
                n121 = call "Enqueue.vi"("Message Data"=w69, "Message"="ShowPanel", "MessageQueue"=w68) -> ("error out"=w66:errorcluster)  [unwired: 7 in, 1 out]
              }
            }
          }
          event User Event {
            n122 = event-data() -> ("ModuleID"=w72:i32, "Data"=w71:variant)  [unwired: 1 in]
            n123 = call <userlib>:"AddressedToThisModule.vi"("ModuleID"=w72, "ModuleAdmin"=w74) -> ("AddressedToThisInstance?"=w75:bool)  [unwired: 8 in, 1 out]
            n124 = case shown="True" w75 {
              tunnel: w71 -> [_ w79]
              tunnel: w73 -> [_ w78]
              tunnel: [_ w76] -> w70
              frame False {
              }
              frame True {
                n125 = call "Enqueue.vi"("Message Data"=w79, "Message"="ReadPathToPlugin", "MessageQueue"=w78) -> ("error out"=w76:errorcluster)  [unwired: 7 in, 1 out]
              }
            }
          }
          event User Event {
            n126 = event-data() -> ("ModuleID"=w85:i32, "Data"=w82:variant)  [unwired: 1 in]
            n127 = call <userlib>:"AddressedToThisModule.vi"("ModuleID"=w85, "ModuleAdmin"=w84) -> ("AddressedToThisInstance?"=w83:bool)  [unwired: 8 in, 1 out]
            n128 = case shown="True" w83 {
              tunnel: w82 -> [_ w89]
              tunnel: w81 -> [_ w87]
              tunnel: [_ w86] -> w80
              frame False {
              }
              frame True {
                n129 = call "Enqueue.vi"("Message Data"=w89, "Message"="WriteEvtConfig", "MessageQueue"=w87) -> ("error out"=w86:errorcluster)  [unwired: 7 in, 1 out]
              }
            }
          }
          event User Event {
            n130 = event-data() -> ("ModuleID"=w94:i32, "Data"=w93:variant)  [unwired: 1 in]
            n131 = call <userlib>:"AddressedToThisModule.vi"("ModuleID"=w94, "ModuleAdmin"=w95) -> ("AddressedToThisInstance?"=w92:bool)  [unwired: 8 in, 1 out]
            n132 = case shown="True" w92 {
              tunnel: w93 -> [_ w99]
              tunnel: w91 -> [_ w98]
              tunnel: [_ w96] -> w90
              frame False {
              }
              frame True {
                n133 = call "Enqueue.vi"("Message Data"=w99, "Message"="ReadEvtConfig", "MessageQueue"=w98) -> ("error out"=w96:errorcluster)  [unwired: 7 in, 1 out]
              }
            }
          }
          event User Event {
            n134 = event-data() -> ("ModuleID"=w102:i32, "Data"=w101:variant)  [unwired: 1 in]
            n135 = call <userlib>:"AddressedToThisModule.vi"("ModuleID"=w102, "ModuleAdmin"=w103) -> ("AddressedToThisInstance?"=w105:bool)  [unwired: 8 in, 1 out]
            n136 = case shown="True" w105 {
              tunnel: [_ w108] -> w104
              tunnel: w101 -> [_ w107]
              tunnel: w100 -> [_ w106]
              frame False {
              }
              frame True {
                n137 = call "Enqueue.vi"("Message Data"=w107, "Message"="WriteTimeArray", "MessageQueue"=w106) -> ("error out"=w108:errorcluster)  [unwired: 7 in, 1 out]
              }
            }
          }
          event User Event {
            n138 = event-data() -> ("ModuleID"=w112:i32, "Data"=w111:variant)  [unwired: 1 in]
            n139 = call <userlib>:"AddressedToThisModule.vi"("ModuleID"=w112, "ModuleAdmin"=w114) -> ("AddressedToThisInstance?"=w115:bool)  [unwired: 8 in, 1 out]
            n140 = case shown="True" w115 {
              tunnel: [_ w118] -> w110
              tunnel: w113 -> [_ w117]
              tunnel: w111 -> [_ w116]
              frame False {
              }
              frame True {
                n141 = call "Enqueue.vi"("Message Data"=w116, "Message"="ReadTimeArray", "MessageQueue"=w117) -> ("error out"=w118:errorcluster)  [unwired: 7 in, 1 out]
              }
            }
          }
          event User Event {
            n142 = event-data() -> ("ModuleID"=w123:i32, "Data"=w124:variant)  [unwired: 1 in]
            n143 = call <userlib>:"AddressedToThisModule.vi"("ModuleID"=w123, "ModuleAdmin"=w122) -> ("AddressedToThisInstance?"=w125:bool)  [unwired: 8 in, 1 out]
            n144 = case shown="True" w125 {
              tunnel: [_ w128] -> w120
              tunnel: w124 -> [_ w127]
              tunnel: w121 -> [_ w126]
              frame False {
              }
              frame True {
                n145 = call "Enqueue.vi"("Message Data"=w127, "Message"="WriteEvtParams", "MessageQueue"=w126) -> ("error out"=w128:errorcluster)  [unwired: 7 in, 1 out]
              }
            }
          }
          event User Event {
            n146 = event-data() -> ("ModuleID"=w132:i32, "Data"=w134:variant)  [unwired: 1 in]
            n147 = call <userlib>:"AddressedToThisModule.vi"("ModuleID"=w132, "ModuleAdmin"=w133) -> ("AddressedToThisInstance?"=w135:bool)  [unwired: 8 in, 1 out]
            n148 = case shown="True" w135 {
              tunnel: [_ w138] -> w130
              tunnel: w134 -> [_ w137]
              tunnel: w131 -> [_ w136]
              frame False {
              }
              frame True {
                n149 = call "Enqueue.vi"("Message Data"=w137, "Message"="ReadEvtParams", "MessageQueue"=w136) -> ("error out"=w138:errorcluster)  [unwired: 7 in, 1 out]
              }
            }
          }
          event User Event {
            n150 = event-data() -> ("ModuleID"=w143:i32, "Data"=w144:variant)  [unwired: 1 in]
            n151 = call <userlib>:"AddressedToThisModule.vi"("ModuleID"=w143, "ModuleAdmin"=w142) -> ("AddressedToThisInstance?"=w145:bool)  [unwired: 8 in, 1 out]
            n152 = case shown="True" w145 {
              tunnel: [_ w148] -> w140
              tunnel: w144 -> [_ w147]
              tunnel: w141 -> [_ w146]
              frame False {
              }
              frame True {
                n153 = call "Enqueue.vi"("Message Data"=w147, "Message"="WriteBusNumber", "MessageQueue"=w146) -> ("error out"=w148:errorcluster)  [unwired: 7 in, 1 out]
              }
            }
          }
          event User Event {
            n154 = event-data() -> ("ModuleID"=w153:i32, "Data"=w154:variant)  [unwired: 1 in]
            n155 = call <userlib>:"AddressedToThisModule.vi"("ModuleID"=w153, "ModuleAdmin"=w152) -> ("AddressedToThisInstance?"=w155:bool)  [unwired: 8 in, 1 out]
            n156 = case shown="True" w155 {
              tunnel: [_ w158] -> w150
              tunnel: w154 -> [_ w157]
              tunnel: w151 -> [_ w156]
              frame False {
              }
              frame True {
                n157 = call "Enqueue.vi"("Message Data"=w157, "Message"="ReadBusNumber", "MessageQueue"=w156) -> ("error out"=w158:errorcluster)  [unwired: 7 in, 1 out]
              }
            }
          }
          event User Event {
            n158 = event-data() -> ("ModuleID"=w163:i32, "Data"=w161:variant)  [unwired: 1 in]
            n159 = call <userlib>:"AddressedToThisModule.vi"("ModuleID"=w163, "ModuleAdmin"=w164) -> ("AddressedToThisInstance?"=w165:bool)  [unwired: 8 in, 1 out]
            n160 = case shown="True" w165 {
              tunnel: [_ w168] -> w160
              tunnel: w162 -> [_ w167]
              tunnel: w161 -> [_ w166]
              frame False {
              }
              frame True {
                n161 = call "Enqueue.vi"("Message Data"=w166, "Message"="GetReportArray", "MessageQueue"=w167) -> ("error out"=w168:errorcluster)  [unwired: 7 in, 1 out]
              }
            }
          }
          event User Event {
            n162 = event-data() -> ("ModuleID"=w173:i32, "Data"=w171:variant)  [unwired: 1 in]
            n163 = call <userlib>:"AddressedToThisModule.vi"("ModuleID"=w173, "ModuleAdmin"=w174) -> ("AddressedToThisInstance?"=w175:bool)  [unwired: 8 in, 1 out]
            n164 = case shown="True" w175 {
              tunnel: [_ w178] -> w170
              tunnel: w172 -> [_ w177]
              tunnel: w171 -> [_ w176]
              frame False {
              }
              frame True {
                n165 = call "Enqueue.vi"("Message Data"=w176, "Message"="GetEvtSignal", "MessageQueue"=w177) -> ("error out"=w178:errorcluster)  [unwired: 7 in, 1 out]
              }
            }
          }
          event Panel Close? {
            # "Hide on external launch"
            # "Discard the event so the QMH can complete"
            # "Called from another module or the QMH"
            n166 = event-data() -> ()  [unwired: 1 in, 1 out]
            n167 = property class="ModuleAdmin.lvclass"(reference=w186) -> ("Accessors:External Launch"=w181:bool)  [unwired: 1 in, 2 out]
            n168 = Bundle By Name(cluster=T3 {"Exit via Stop Module Req?"=FALSE, "Wait for Module to stop?"=FALSE, "ModuleAdmin"=refnum} ("Stop Argument"), "Wait for Module to stop?"=FALSE, "Exit via Stop Module Req?"=TRUE) -> (w187:T3)
            n169 = Select(t="HidePanel", s=w181, f="Exit" ("Message")) -> (s? t:f=w183:string)
            n170 = call "Enqueue.vi"("Message Data"=w187, "Message"=w183, "MessageQueue"=w192) -> ("error out"=w190:errorcluster)  [unwired: 7 in, 1 out]
            n171 = event-data("Discard?"=TRUE) -> ()  [unwired: 1 in, 1 out]
          }
        }
        n172 = call "ErrorHandler.vi"("error in (no error)"=w32, "MessageQueue"=w30) -> ("error out"=w31:errorcluster)  [unwired: 8 in, 1 out]
      }
    }
    frame Error {
      n173 = property class="ModuleAdmin.lvclass"(reference=w506) -> (reference out=w505:refnum<class "ModuleAdmin.lvclass">, "Accessors:CloneRegRef"=w503:refnum<data-value>, "Accessors:Module ID"=w502:i32)  [unwired: 1 in, 1 out]
      n174 = call <userlib>:"Remove.vi"("Module ID"=w502, "CloneRegRef"=w503) -> ("error out"=w508:errorcluster)  [unwired: 7 in, 2 out]
      n175 = flat-sequence {
        tunnel: w509 -> [w512]
        tunnel: w508 -> [_]
        tunnel: [w510] -> w507
        frame #0 {
          w511 = T11 2 items=["no dialog", "OK message", "continue or stop message", "OK message + warnings", "continue/stop + warnings"] ("type of dialog (OK msg:1)")
          n176 = call <vilib>:"Simple Error Handler.vi"("type of dialog (OK msg:1)"=w511, "error in (no error)"=w512) -> ("error out"=w510:errorcluster)  [unwired: 3 in, 4 out]
        }
      }
    }
  }
  n177 = call "DestroyClone.vi"("error in (no error)"=w8, "Exit via Stop Module Req?"=w4, "Wait for Module to stop?"=w5, "ModuleAdmin"=w6) -> ("error out"=w7:errorcluster, "External Launch"=w3:bool)  [unwired: 5 in, 1 out]
  n178 = Release Queue(queue=w1, error in (no error)=w7) -> (error out=w2:errorcluster)  [unwired: 1 in, 2 out]
  "error out" <- w2
  n179 = case shown="True" w3 {
    tunnel: w2 -> [_ w514]
    frame False {
    }
    frame True {
      n180 = control-ref of="This VI"() -> (w513:refnum<vi>)
      n181 = case shown="Error" w514 {
        tunnel: w513 -> [w515 w516]
        frame No Error {
          n182 = invoke class="VI" method="FP.Close"(reference=w515) -> ()  [unwired: 2 in, 3 out]
        }
        frame Error {
          n183 = invoke class="VI" method="FP.Open"(reference=w516, "Activate"=TRUE ("Activate?")) -> ()  [unwired: 3 in, 5 out]
        }
      }
    }
  }
